vi "Configure Stray Light Constant.vi"(8 "error in (no error)":errorcluster, 10 "Stray Light Constant (0)":dbl, 11 "VISA resource name":refnum<visa-resource-name>) -> (0 "error out":errorcluster, 3 "VISA resource name out":refnum<visa-resource-name>)   [LabVIEW 2021, in "Ocean Optics 2000 4000.lvlib"]
doc: "Configures the stray light calibration constant. This setting is saved in the instrument EEPROM. \n\n<b>Note:</b>\nThis VI is reserved for advanced users. Changing these values may cause the spectrometer to be wrongly calibrated.\nConsult support from Ocean Optics before running this VI!"
uses:
  <instrlib>/Ocean Optics 2000 4000/Ocean Optics 2000 4000.lvlib
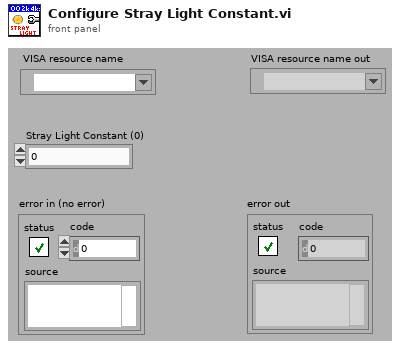
[diagram p1: front panel]
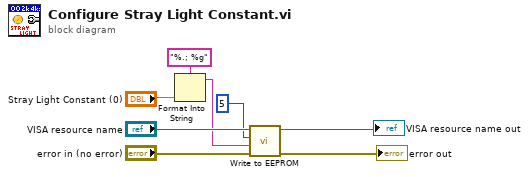
[diagram p0: block diagram]
diagram:
  n1 = Format Into String(format string="%.; %g", "Stray Light Constant (0)") -> (resulting string=w2:string)  [unwired: 2 in, 1 out]
  n2 = call <instrlib>:"Write to EEPROM.vi"("error in (no error)"="error in (no error)", "15 Byte ASCII"=w2, "EEPROM Index"=u8 5, "VISA resource name"="VISA resource name") -> ("error out"=→"error out":errorcluster, "VISA resource name out"=→"VISA resource name out":refnum<visa-resource-name>)  [unwired: 6 out]
